vi "mes~产品加工参数采集.vi"(8 "error in (no error)":errorcluster caption="错误输入（无错误）", 9 "采集项":string[](array[string]), 11 "测试结果":string caption="测试结果:") -> (0 "error out":errorcluster caption="错误输出", 2 "加工参数采集成功":bool)   [LabVIEW 2015]
uses:
  ctl/SendproductParaColloctUniversal.ctl
  ctl/ReceiveproductParaColloctUniversal.ctl
  Global.vi
panel:
  in  "Headers":string[][](array[string])=[["Content-Type", "text/xml;charset=UTF-8"], ["SOAPAction", "\"http://tempuri.org/IUserRightVerifyServiceImpl/UserRightVerify\""], ["Connection", "Keep-Alive"], ["User-Agent", "Apache-HttpClient/4.1.1 (java 1.5)"]]
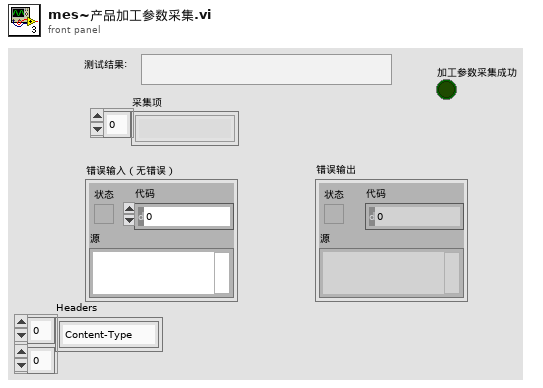
[diagram p1: front panel]
types:
  T1 = typedef "SendproductParaColloctUniversal.ctl" = cluster{"#attributes":cluster{"xmlns:soapenv":string, "xmlns:tem":string, "xmlns:cal":string}, "soapenv:Header":string, "soapenv:Body":cluster{"tem:productParaColloctUniversal":cluster{"tem:vo":cluster{"cal:completeQty":string, "cal:equipNum":string, "cal:identification":string, "cal:productType":string, "cal:qualityStatus":string, "cal:recordDate":string, "cal:siteCode":string, "cal:tagData":cluster{"cal:TagDataV0":cluster{"cal:tagCode":string, "cal:tagValue":string}[]}, "cal:testOrderNum":string, "cal:userName":string}}}}
  T2 = cluster{"接口地址(URL)":string, "设备编号(equipNum)":string, "站点名称(siteCode)":string, "生产类型(productType)":string, "试验单号(testOrderNum)":string}
  T3 = typedef "ReceiveproductParaColloctUniversal.ctl" = cluster{"#attributes":cluster{"xmlns:s":string}, "s:Body":cluster{"productParaColloctUniversalResponse":cluster{"#attributes":cluster{"xmlns":string}, "productParaColloctUniversalResult":cluster{"#attributes":cluster{"xmlns:a":string, "xmlns:i":string}, "a:ErrorCode":string, "a:ErrorMessage":string, "a:Success":string}}}}
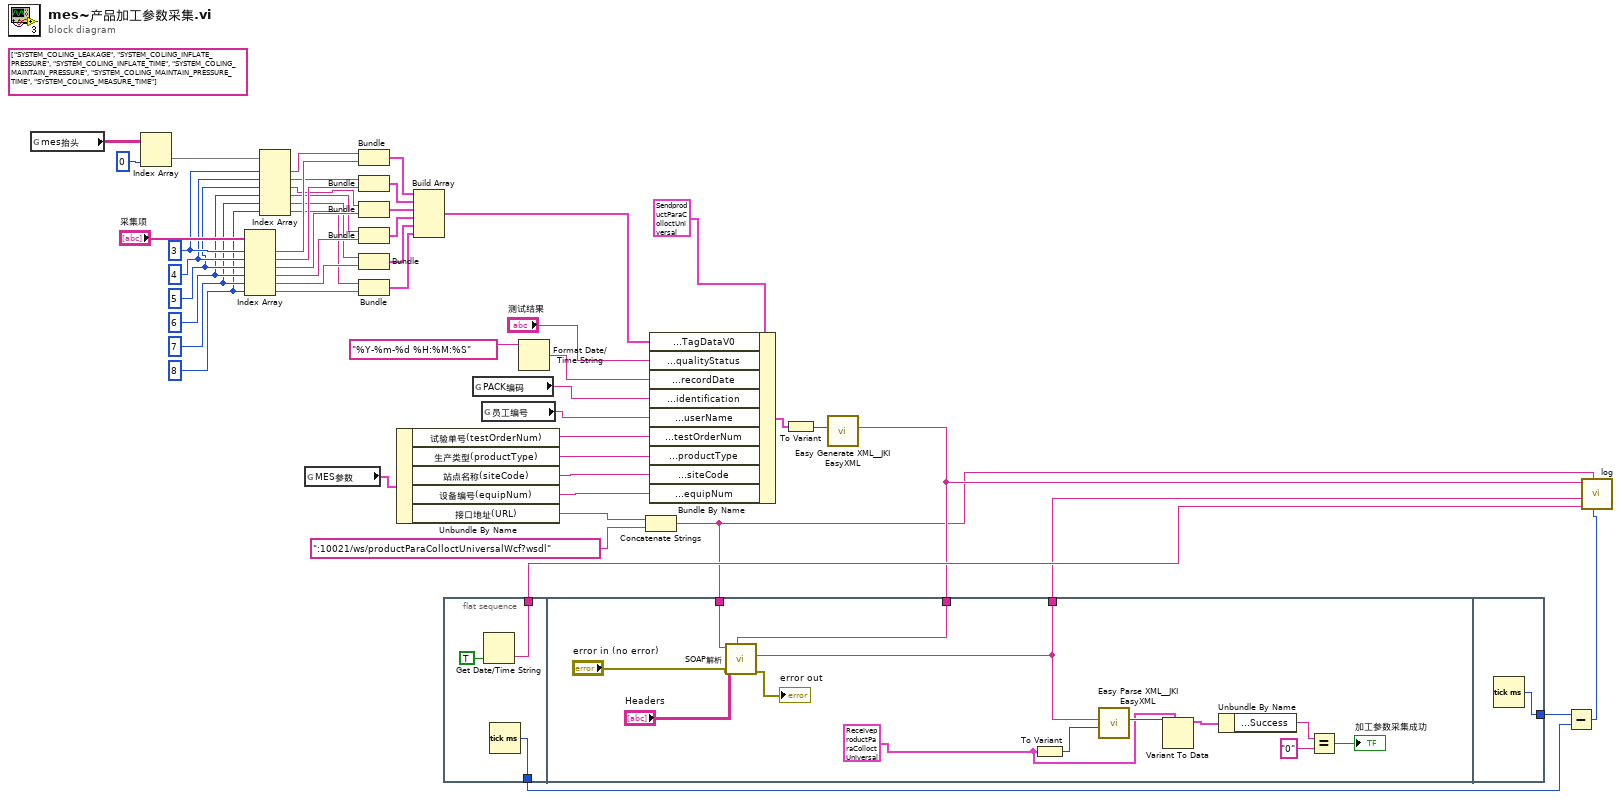
[diagram p0: block diagram]
diagram:
  (unwired) string[] ["SYSTEM_COLING_LEAKAGE", "SYSTEM_COLING_INFLATE_PRESSURE", "SYSTEM_COLING_INFLATE_TIME", "SYSTEM_COLING_MAINTAIN_PRESSURE", "SYSTEM_COLING_MAINTAIN_PRESSURE_TIME", "SYSTEM_COLING_MEASURE_TIME"]
  w9 = 8 ("索引")
  w11 = 7 ("索引")
  w12 = 6 ("索引")
  w13 = 5 ("索引")
  w14 = 4 ("索引")
  w15 = 3 ("索引")
  n1 = global read "Global.vi" "mes抬头"() -> (w17:string[][])
  n2 = Index Array(array=w17, index (col)=0 ("禁用的索引 (列)")) -> (element=w16:string[])  [unwired: 1 in]
  n3 = Index Array(array="采集项", index #1=w15, index #2=w14, index #3=w13, index #4=w12, index #5=w11, index #6=w9) -> (element #1=w35:string, element #2=w34:string, element #3=w30:string, element #4=w28:string, element #5=w26:string, element #6=w24:string)
  n4 = Index Array(array=w16, index #1=w15, index #2=w14, index #3=w13, index #4=w12, index #5=w11, index #6=w9) -> (element #1=w33:string, element #2=w32:string, element #3=w31:string, element #4=w29:string, element #5=w27:string, element #6=w25:string)
  n5 = global read "Global.vi" "MES参数"() -> (w47:T2)
  n6 = Bundle("String"=w33, "值解析"=w35) -> (w43:cluster{"String":string, "值解析":string})  [unwired: 1 in]
  n7 = Bundle("String"=w32, "值解析"=w34) -> (w23:cluster{"String":string, "值解析":string})  [unwired: 1 in]
  n8 = Bundle("String"=w31, "值解析"=w30) -> (w22:cluster{"String":string, "值解析":string})  [unwired: 1 in]
  n9 = Bundle("String"=w29, "值解析"=w28) -> (w21:cluster{"String":string, "值解析":string})  [unwired: 1 in]
  n10 = Bundle("String"=w27, "值解析"=w26) -> (w20:cluster{"String":string, "值解析":string})  [unwired: 1 in]
  n11 = Bundle("String"=w25, "值解析"=w24) -> (w10:cluster{"String":string, "值解析":string})  [unwired: 1 in]
  n12 = Unbundle By Name(w47) -> ("试验单号(testOrderNum)"=w42:string, "生产类型(productType)"=w44:string, "站点名称(siteCode)"=w48:string, "设备编号(equipNum)"=w49:string, "接口地址(URL)"=w46:string)
  n13 = Build Array(w43, w23, w22, w21, w20, w10) -> (w19:cluster{"String":string, "值解析":string}[])
  n14 = flat-sequence {
    tunnel: [w53] -> w7
    tunnel: [w52] -> w6
    tunnel: w4 -> [w57]
    tunnel: [w56] -> w3
    tunnel: w1 -> [w58]
    tunnel: [w68] -> w8
    frame #0 {
      n15 = Get Date/Time String(want seconds? (F)=TRUE ("需要秒？(F)")) -> (time string=w52:string)  [unwired: 2 in, 1 out]
      n16 = Tick Count (ms)() -> (millisecond timer value=w53:u32)
    }
    frame #1 {
      w61 = T3 {"#attributes"={"xmlns:s"="http://schemas.xmlsoap.org/soap/envelope/"}, "s:Body"={"productParaColloctUniversalResponse"={"#attributes"={"xmlns"="http://tempuri.org/"}, "productParaColloctUniversalResult"={"#attributes"={"xmlns:a"="http://schemas.datacontract.org/2004/07/EdgeUtility", "xmlns:i"="http://www.w3.org/2001/XMLSchema-instance"}, "a:ErrorCode"="", "a:ErrorMessage"="", "a:Success"=""}}}} ("s:Envelope")
      n17 = call "SOAP解析.vi"("DATA"=w57, "错误输入（无错误）"="error in (no error)", "Headers"="Headers", "URL"=w58) -> ("错误输出"=→"error out":errorcluster, "body"=w56:string)  [unwired: 5 in, 1 out]
      n18 = To Variant(anything=w61) -> (Variant=w67:variant)
      n19 = call <vilib>:"Easy Parse XML__JKI EasyXML.vi"("LabVIEW Data (Type)"=w67, "XML String"=w56) -> ("LabVIEW Data"=w66:variant)  [unwired: 8 in, 1 out]
      n20 = Variant To Data(type=w61, Variant=w66) -> (data=w65:T3)  [unwired: 1 in, 1 out]
      n21 = Unbundle By Name(w65) -> ("s:Body.productParaColloctUniversalResponse.productParaColloctUniversalResult.a:Success"=w64:string)
      n22 = Equal?(x=w64, y="0") -> (x = y?=→"加工参数采集成功":bool)
    }
    frame #2 {
      n23 = Tick Count (ms)() -> (millisecond timer value=w68:u32)
    }
  }
  n24 = global read "Global.vi" "PACK编码"() -> (w40:string)
  n25 = global read "Global.vi" "员工编号"() -> (w41:string)
  n26 = Format Date/Time String(time format string (%c)="%Y-%m-%d %H:%M:%S" ("时间格式字符串(%c)")) -> (date/time string=w38:string)  [unwired: 2 in]
  n27 = Concatenate Strings(w46, ":10021/ws/productParaColloctUniversalWcf?wsdl") -> (w1:string)
  n28 = Bundle By Name(cluster=T1 {"#attributes"={"xmlns:soapenv"="http://schemas.xmlsoap.org/soap/envelope/", "xmlns:tem"="http://tempuri.org/", "xmlns:cal"="http://schemas.datacontract.org/2004/07/CalbProductParaColloctUniversalService"}, "soapenv:Header"="", "soapenv:Body"={"tem:productParaColloctUniversal"={"tem:vo"={"cal:completeQty"="", "cal:equipNum"="", "cal:identification"="", "cal:productType"="", "cal:qualityStatus"="", "cal:recordDate"="", "cal:siteCode"="", "cal:tagData"={"cal:TagDataV0"=[]}, "cal:testOrderNum"="", "cal:userName"=""}}}} ("soapenv:Envelope"), "soapenv:Body.tem:productParaColloctUniversal.tem:vo.cal:tagData.cal:TagDataV0"=w19, "soapenv:Body.tem:productParaColloctUniversal.tem:vo.cal:qualityStatus"="测试结果", "soapenv:Body.tem:productParaColloctUniversal.tem:vo.cal:recordDate"=w38, "soapenv:Body.tem:productParaColloctUniversal.tem:vo.cal:identification"=w40, "soapenv:Body.tem:productParaColloctUniversal.tem:vo.cal:userName"=w41, "soapenv:Body.tem:productParaColloctUniversal.tem:vo.cal:testOrderNum"=w42, "soapenv:Body.tem:productParaColloctUniversal.tem:vo.cal:productType"=w44, "soapenv:Body.tem:productParaColloctUniversal.tem:vo.cal:siteCode"=w48, "soapenv:Body.tem:productParaColloctUniversal.tem:vo.cal:equipNum"=w49) -> (w51:T1)
  n29 = To Variant(anything=w51) -> (Variant=w50:variant)
  n30 = call <vilib>:"Easy Generate XML__JKI EasyXML.vi"("LabVIEW Data"=w50) -> ("XML String"=w4:string)  [unwired: 9 in, 1 out]
  n31 = Subtract(x=w8, y=w7) -> (x-y=w5:u32)
  n32 = call "log.vi"("接口耗时"=w5, "URL"=w1, "StartTime"=w6, "响应报文"=w3, "发送报文"=w4) -> ()  [unwired: 7 in]
